vi "load class.vi"(8 "error in":errorcluster, 9 "available class paths":path[](array[path]), 10 "available class names":string[](array[string]), 11 "Class Name":string) -> (0 "error out":errorcluster, 3 "Object Out":refnum<class>)   [LabVIEW 2025, in "CEF.lvlib"]
doc: "Attempts to load a class, by name, either from memory or from disk. First it tries the exact name in memory. Then it tries the filename on disk. Then it tries an approximate match of all VIs in memory.Copyright 2017 National Instruments Corporation\n\nLicensed under the Apache License, Version 2.0 (the \"License\"); you may not use this file except in compliance with the License. You may obtain a copy of the License at http://www.apache.org/licenses/LICENSE-2.0\nUnless required by applicable law or agreed to in writing, software distributed under the License is distributed on an \"AS IS\" BASIS, WITHOUT WARRANTIES OR CONDITIONS OF ANY KIND, either express or implied. See the License for the specific language governing permissions and limitations under the License."
uses:
  CEF.lvlib
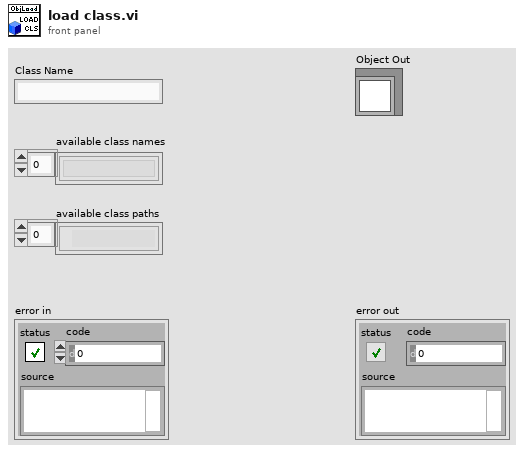
[diagram p1: front panel]
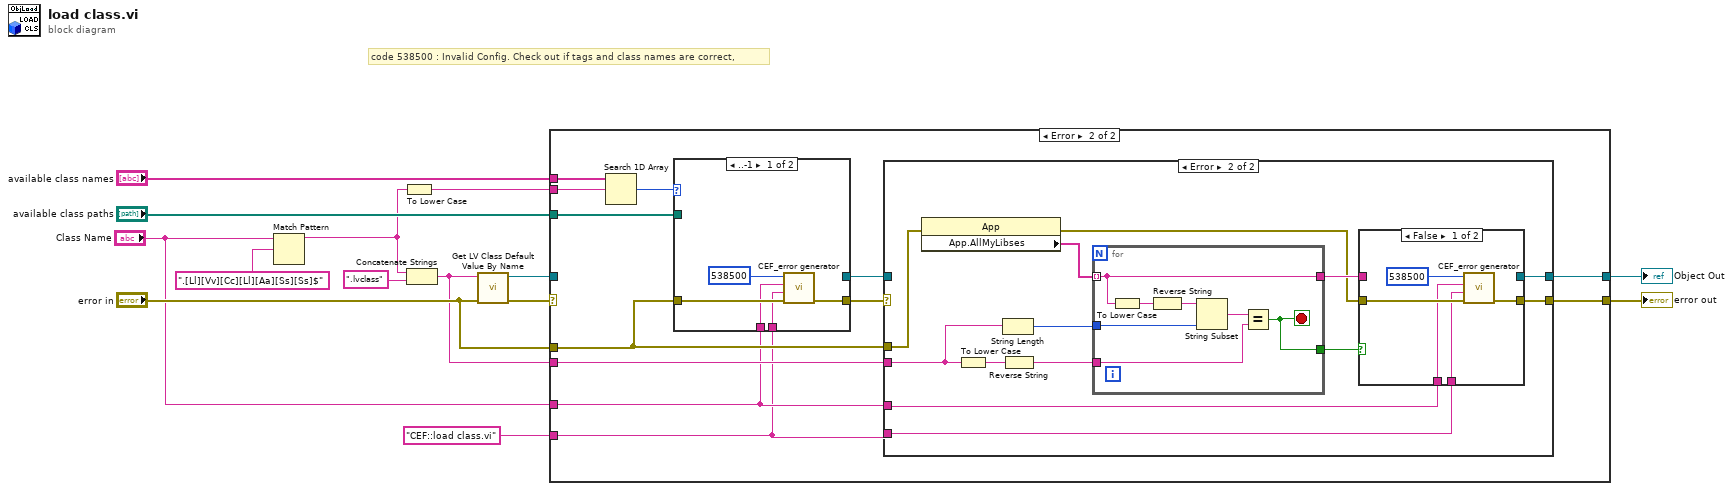
[diagram p0: block diagram]
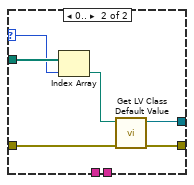
[diagram p3: hidden frame]
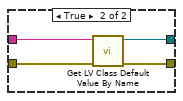
[diagram p5: hidden frame]
diagram:
  # "code 538500 : Invalid Config. Check out if tags and class names are correct,"
  n1 = Match Pattern(string="Class Name", regular expression=".[Ll][Vv][Cc][Ll][Aa][Ss][Ss]$") -> (before substring=w3:string)  [unwired: 1 in, 3 out]
  n2 = To Lower Case(string=w3) -> (all lower case string=w9:string)
  n3 = Concatenate Strings(w3, ".lvclass" ("string")) -> (w5:string)
  n4 = call <vilib>:"Get LV Class Default Value By Name.vi"("error in (no error)"="error in", "class name"=w5) -> ("error out"=w8:errorcluster, "object"=w6:refnum<class>)  [unwired: 8 in]
  n5 = case shown="Error" w8 {
    selector: w8 -> [w15 _]
    tunnel: [w16 w28] -> w12
    tunnel: w6 -> [w16 _]
    tunnel: [w15 w27] -> w13
    tunnel: "error in" -> [_ w26]
    tunnel: w9 -> [_ w22]
    tunnel: "available class names" -> [_ w23]
    tunnel: "Class Name" -> [_ w18]
    tunnel: "available class paths" -> [_ w20]
    tunnel: w5 -> [_ w19]
    tunnel: "CEF::load class.vi" -> [_ w17]
    frame No Error {
    }
    frame Error {
      n6 = Search 1D Array(1D array=w23, element=w22) -> (index of element=w21:i32)  [unwired: 1 in]
      n7 = case shown="..-1" w21 {
        selector: w21 -> [_ w35]
        tunnel: w26 -> [w31 w39]
        tunnel: [w32 w38] -> w25
        tunnel: [_ w37] -> w24
        tunnel: w20 -> [_ w36]
        tunnel: w17 -> [w30 _]
        tunnel: w18 -> [w29 _]
        frame ..-1 {
          n8 = call "CEF_error generator.vi"("error in"=w31, "source"=w30, "append error message"=w29, "error code (0)"=538500) -> ("error out"=w32:errorcluster)  [unwired: 5 in]
        }
        frame 0.. {
          n9 = Index Array(array=w36, index=w35) -> (element=w34:path)
          n10 = call <vilib>:"Get LV Class Default Value.vi"("error in (no error)"=w39, "class path"=w34) -> ("error out"=w38:errorcluster, "object"=w37:refnum<class>)  [unwired: 8 in]
        }
      }
      n11 = case shown="Error" w25 {
        selector: w25 -> [w41 _]
        tunnel: [w40 w47] -> w28
        tunnel: [w41 w48] -> w27
        tunnel: w26 -> [_ w54]
        tunnel: w24 -> [w40 _]
        tunnel: w19 -> [_ w46]
        tunnel: w18 -> [_ w45]
        tunnel: w17 -> [_ w42]
        frame No Error {
        }
        frame Error {
          n12 = property class="App"(error in=w54) -> (error out=w49:errorcluster, "App.AllMyLibses"=w53:string[])  [unwired: 1 in, 1 out]
          n13 = To Lower Case(string=w46) -> (all lower case string=w44:string)
          n14 = String Length(string=w46) -> (length=w52:i32)
          n15 = Reverse String(1:w44) -> (0:w43:string)
          n16 = for {
            tunnel: w53 -> [w66] mode=indexing
            tunnel: w43 -> [w64]
            tunnel: w52 -> [w69]
            tunnel: [w66] -> w51
            tunnel: [w68] -> w50
            stop <- w68 stop-if-true
            n17 = To Lower Case(string=w66) -> (all lower case string=w67:string)
            n18 = Reverse String(1:w67) -> (0:w70:string)
            n19 = String Subset(string=w70, length (rest)=w69) -> (substring=w65:string)  [unwired: 1 in]
            n20 = Equal?(x=w65, y=w64) -> (x = y?=w68:bool)
          }
          n21 = case shown="False" w50 {
            tunnel: w51 -> [_ w63]
            tunnel: w49 -> [w57 w62]
            tunnel: [w58 w61] -> w48
            tunnel: [_ w60] -> w47
            tunnel: w45 -> [w56 _]
            tunnel: w42 -> [w55 _]
            frame False {
              n22 = call "CEF_error generator.vi"("error in"=w57, "source"=w55, "append error message"=w56, "error code (0)"=538500) -> ("error out"=w58:errorcluster)  [unwired: 5 in]
            }
            frame True {
              n23 = call <vilib>:"Get LV Class Default Value By Name.vi"("error in (no error)"=w62, "class name"=w63) -> ("error out"=w61:errorcluster, "object"=w60:refnum<class>)  [unwired: 8 in]
            }
          }
        }
      }
    }
  }
  "error out" <- w13
  "Object Out" <- w12
